vi "Get-Set Reserved Keywords.vi"(6 "Get (F)/Set":bool, 8 "Error In":errorcluster, 9 "Formula Interpreter Path":path, 11 "Reserved Keywords":string[](array[string])) -> (0 "Error Out":errorcluster, 1 "Formula Interpreter Path":path, 3 "Reserved Keywords":string[](array[string]))   [LabVIEW 2021, in "Formula.lvlib"]
uses:
  Formula.lvlib
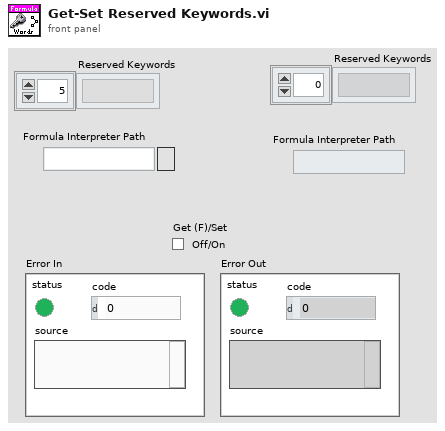
[diagram p1: front panel]
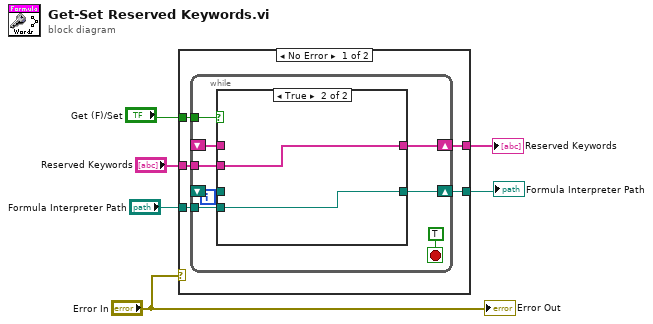
[diagram p0: block diagram]
diagram:
  n1 = case shown="No Error" "Error In" {
    tunnel: "Get (F)/Set" -> [w11 _]
    tunnel: [w10 _] -> w5
    tunnel: "Reserved Keywords" -> [w9 _]
    tunnel: "Formula Interpreter Path" -> [w8 _]
    tunnel: [w7 _] -> w1
    frame No Error {
      n2 = while {
        tunnel: w11 -> [w18]
        shift-right: [w17] -> w10
        shift-left: _ -> [w15]
        tunnel: w9 -> [w16]
        shift-right: [w13] -> w7
        shift-left: _ -> [w12]
        tunnel: w8 -> [w14]
        stop <- TRUE stop-if-true
        n3 = case shown="True" w18 {
          tunnel: [w21 w23] -> w17
          tunnel: w16 -> [_ w23]
          tunnel: w15 -> [w21 _]
          tunnel: w14 -> [_ w22]
          tunnel: [w20 w22] -> w13
          tunnel: w12 -> [w20 _]
          frame False {
          }
          frame True {
          }
        }
      }
    }
    frame Error {
    }
  }
  "Reserved Keywords" <- w5
  "Formula Interpreter Path" <- w1
  "Error Out" <- "Error In"
